vi "New Picture.vi"(7 "xwpfParagraph Type":refnum<class "xwpfParagraph.lvclass">, 8 "error in (no error)":errorcluster, 10 "Picture File Path":path, 11 "Paragraph.Ref":refnum<k24>) -> (0 "error out":errorcluster, 3 "xwpfParagraph out":refnum<class "xwpfParagraph.lvclass">)   [LabVIEW 2017, in "Word_Specific.lvlib" / "xwpfParagraph.lvclass"]
uses:
  xwpfParagraph.lvclass
  C:/Users/Neo/Desktop/Dev_Tools_BR/LabVIEW_NPOI/src/lib/NPOI 2.1.1/NPOI.OOXML.dll
  lib/NPOI 2.1.1/NPOI.OOXML.dll
  xwpfParagraph.lvclass/xwpfParagraph.ctl
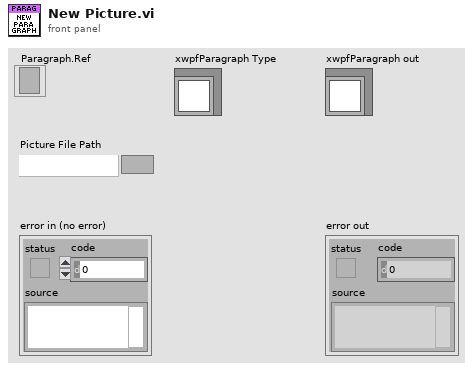
[diagram p1: front panel]
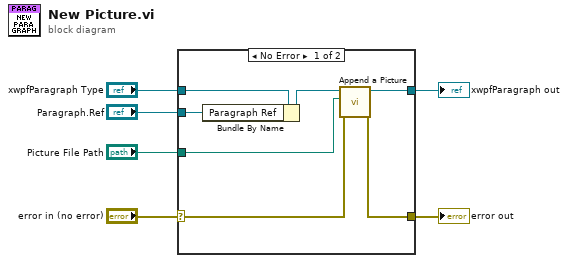
[diagram p0: block diagram]
diagram:
  n1 = case shown="No Error" "error in (no error)" {
    selector: "error in (no error)" -> [w11 w15]
    tunnel: [w12 w15] -> w5
    tunnel: [w13 w14] -> w3
    tunnel: "xwpfParagraph Type" -> [w10 w14]
    tunnel: "Paragraph.Ref" -> [w8 _]
    tunnel: "Picture File Path" -> [w7 _]
    frame No Error {
      n2 = Bundle By Name(cluster=w10, "Paragraph Ref"=w8) -> (w9:refnum<class "xwpfParagraph.lvclass">)
      n3 = call "Append a Picture.vi"("error in (no error)"=w11, "Picture File Path"=w7, "xwpfParagraph in"=w9) -> ("error out"=w12:errorcluster, "xwpfParagraph out"=w13:refnum<class "xwpfParagraph.lvclass">)  [unwired: 7 in]
    }
    frame Error {
    }
  }
  "error out" <- w5
  "xwpfParagraph out" <- w3
